vi "Convert Event String to Enum.vi"(11 "Event String":string) -> (3 "Event":T1)   [LabVIEW 2015, in "NI_AWS_S3.lvlib"]
doc: "Convert the Permission represented as a String to the Enum typedef representation."
uses:
  NI_AWS_S3.lvlib
  Event.ctl
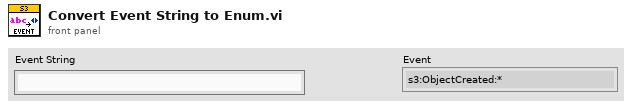
[diagram p1: front panel]
types:
  T1 = typedef "NI_AWS_S3.lvlib/Event.ctl" = enum16{"s3:ObjectCreated:*", "s3:ObjectCreated:Put", "s3:ObjectCreated:Post", "s3:ObjectCreated:Copy", "s3:ObjectCreated:CompleteMultipartUpload", "s3:ObjectRemoved:*", "s3:ObjectRemoved:Delete", "s3:ObjectRemoved:DeleteMarkerCreated", "s3:ReducedRedundancyLostObject"}
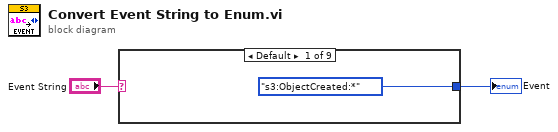
[diagram p0: block diagram]
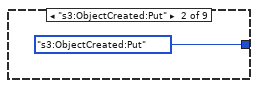
[diagram p2: hidden frame]
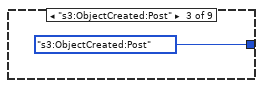
[diagram p3: hidden frame]
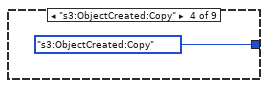
[diagram p4: hidden frame]
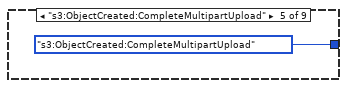
[diagram p5: hidden frame]
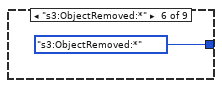
[diagram p6: hidden frame]
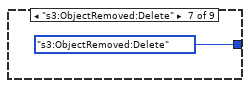
[diagram p7: hidden frame]
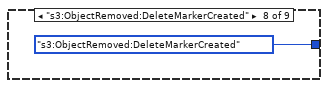
[diagram p8: hidden frame]
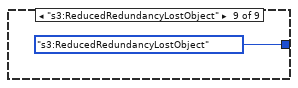
[diagram p9: hidden frame]
diagram:
  n1 = case shown="Default" "Event String" {
    tunnel: [Event."s3:ObjectCreated:*" ("Event") Event."s3:ObjectCreated:Put" ("Event") Event."s3:ObjectCreated:Post" ("Event") Event."s3:ObjectCreated:Copy" ("Event") Event."s3:ObjectCreated:CompleteMultipartUpload" ("Event") Event."s3:ObjectRemoved:*" ("Event") Event."s3:ObjectRemoved:Delete" ("Event") Event."s3:ObjectRemoved:DeleteMarkerCreated" ("Event") Event."s3:ReducedRedundancyLostObject" ("Event")] -> w1
    frame Default {
    }
    frame "s3:ObjectCreated:Put" {
    }
    frame "s3:ObjectCreated:Post" {
    }
    frame "s3:ObjectCreated:Copy" {
    }
    frame "s3:ObjectCreated:CompleteMultipartUpload" {
    }
    frame "s3:ObjectRemoved:*" {
    }
    frame "s3:ObjectRemoved:Delete" {
    }
    frame "s3:ObjectRemoved:DeleteMarkerCreated" {
    }
    frame "s3:ReducedRedundancyLostObject" {
    }
  }
  "Event" <- w1
